vi "tearDown.vi"(8 "error in (no error)":errorcluster, 11 "reference in":refnum<class "Disabled Custom Device.lvclass">) -> (0 "error out":errorcluster, 3 "reference out":refnum<class "Disabled Custom Device.lvclass">)   [LabVIEW 2020, in "Disabled Custom Device.lvclass"]
doc: "tearDown runs after the test method has completed. Use this method to clean up any operations or references that were opened by setUp or the test method. Unit tests should be independent of other unit tests so this VI should ensure that the next test can run in a 'clean' test environment."
uses:
  Disabled Custom Device.lvclass
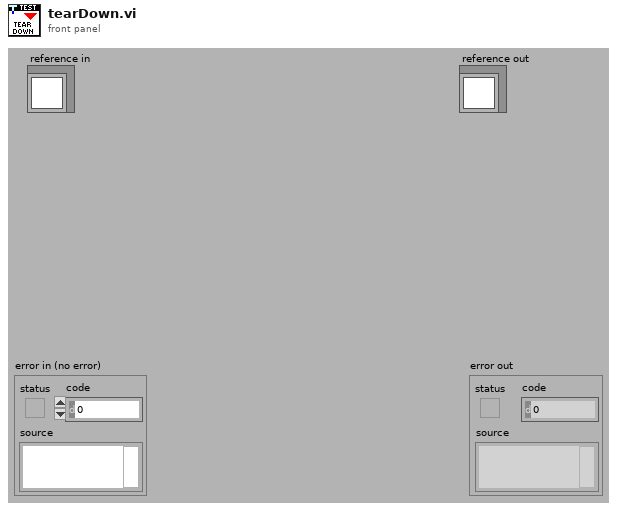
[diagram p1: front panel]
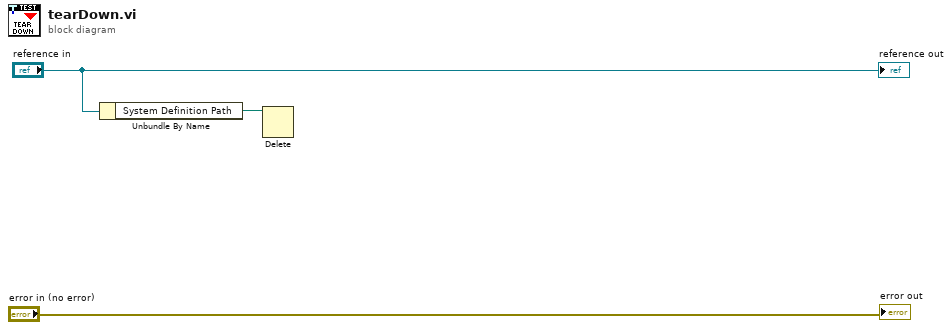
[diagram p0: block diagram]
diagram:
  n1 = Unbundle By Name("reference in") -> ("System Definition Path"=w1:path)
  n2 = Delete(path (use dialog)=w1) -> ()  [unwired: 4 in, 3 out]
  "error out" <- "error in (no error)"
  "reference out" <- "reference in"
